vi "Wait for Event.vi"(8 "error in (no error)":errorcluster, 10 "timeout in ms (-1)":i32, 11 "WAMP Client in":refnum<class "WAMP Client.lvclass">) -> (0 "error out":errorcluster, 1 "timed out?":bool, 2 "WAMP Event":T1, 3 "WAMP Client out":refnum<class "WAMP Client.lvclass">)   [LabVIEW 2020, in "wamplv.lvlib" / "WAMP Client.lvclass"]
doc: "Waits for a WAMP publication event"
uses:
  WAMP Client.lvclass
  TypeDef/Event Payload.ctl
  WAMP Client.lvclass/WAMP Client.ctl
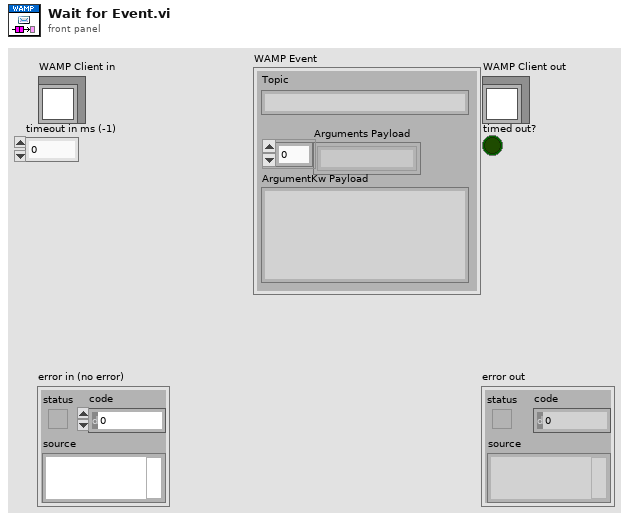
[diagram p1: front panel]
types:
  T1 = typedef "wamplv.lvlib/WAMP Client.lvclass/Event Payload.ctl" = cluster{"Arguments Payload":string[], "ArgumentKw Payload":string, "Topic":string}
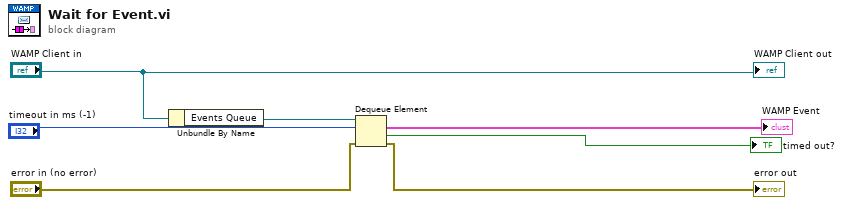
[diagram p0: block diagram]
diagram:
  n1 = Unbundle By Name("WAMP Client in") -> ("Events Queue"=w6:refnum<queue>)
  n2 = Dequeue Element(queue=w6, timeout in ms (-1)="timeout in ms (-1)", error in (no error)="error in (no error)") -> (element=→"WAMP Event":T1, timed out?=→"timed out?":bool, error out=→"error out":errorcluster)  [unwired: 1 out]
  "WAMP Client out" <- "WAMP Client in"
